vi "BuildCmdString.vi"(0 "Reply data 1":u16(ring)=1001 items=["no data"=0, "XYZ position(Command)[rad]"=1, "Joint position(Command)[rad]"=2, "Motor pulse position(Command)"=3, "XYZ position(Feedback)[rad]"=7, "Joint position(Feedback)[rad]"=8, "Motor pulse position(Feedback)"=9, "Current command[0.1%]"=10, "Current feedback[0.1%]"=11, "Robot information"=12, "Position droop"=13, "Speed(Commond)[rpm]"=14, "Speed(Feedback)[rpm]"=15, "Axis load level[%]"=16, "Encoder temperature[C]"=17, "Encoder misscount"=18, "Motor voltage[V]"=19, "Regeneration level[%]"=20, "Tolerable command+[0.1%]"=21, "Tolerable command-[0.1%]"=22, "RMS current[0.1%]"=23, "Force sensor current position"=101, "Force sensor current position(after)"=102, "Force sensor current position(before)"=103, "Position command of the force sensor correction"=104, "COL presumed torque[0.1%]"=111, "COL thershold+[0.1%]"=112, "COL thershold-[0.1%]"=113, "XYZ position(Command)[deg]"=1001, "Joint position(Command)[deg]"=1002, "XYZ position(Feedback)[deg]"=1007, "Joint position(Feedback)[deg]"=1008, "Current command[A]"=1010, "Current feedback[A]"=1011, "Tolerable command+[A]"=1012, "Tolerable command-[A]"=1013, "RMS current[A]"=1014], 1 "Input signal number":u16 max=32767, 2 "Reply data 2":u16(ring)=1002 items=["no data"=0, "XYZ position(Command)[rad]"=1, "Joint position(Command)[rad]"=2, "Motor pulse position(Command)"=3, "XYZ position(Feedback)[rad]"=7, "Joint position(Feedback)[rad]"=8, "Motor pulse position(Feedback)"=9, "Current command[0.1%]"=10, "Current feedback[0.1%]"=11, "Robot information"=12, "Position droop"=13, "Speed(Commond)[rpm]"=14, "Speed(Feedback)[rpm]"=15, "Axis load level[%]"=16, "Encoder temperature[C]"=17, "Encoder misscount"=18, "Motor voltage[V]"=19, "Regeneration level[%]"=20, "Tolerable command+[0.1%]"=21, "Tolerable command-[0.1%]"=22, "RMS current[0.1%]"=23, "Force sensor current position"=101, "Force sensor current position(after)"=102, "Force sensor current position(before)"=103, "Position command of the force sensor correction"=104, "COL presumed torque[0.1%]"=111, "COL thershold+[0.1%]"=112, "COL thershold-[0.1%]"=113, "XYZ position(Command)[deg]"=1001, "Joint position(Command)[deg]"=1002, "XYZ position(Feedback)[deg]"=1007, "Joint position(Feedback)[deg]"=1008, "Current command[A]"=1010, "Current feedback[A]"=1011, "Tolerable command+[A]"=1012, "Tolerable command-[A]"=1013, "RMS current[A]"=1014], 3 "Reply data 3":u16(ring)=102 items=["no data"=0, "XYZ position(Command)[rad]"=1, "Joint position(Command)[rad]"=2, "Motor pulse position(Command)"=3, "XYZ position(Feedback)[rad]"=7, "Joint position(Feedback)[rad]"=8, "Motor pulse position(Feedback)"=9, "Current command[0.1%]"=10, "Current feedback[0.1%]"=11, "Robot information"=12, "Position droop"=13, "Speed(Commond)[rpm]"=14, "Speed(Feedback)[rpm]"=15, "Axis load level[%]"=16, "Encoder temperature[C]"=17, "Encoder misscount"=18, "Motor voltage[V]"=19, "Regeneration level[%]"=20, "Tolerable command+[0.1%]"=21, "Tolerable command-[0.1%]"=22, "RMS current[0.1%]"=23, "Force sensor current position"=101, "Force sensor current position(after)"=102, "Force sensor current position(before)"=103, "Position command of the force sensor correction"=104, "COL presumed torque[0.1%]"=111, "COL thershold+[0.1%]"=112, "COL thershold-[0.1%]"=113, "XYZ position(Command)[deg]"=1001, "Joint position(Command)[deg]"=1002, "XYZ position(Feedback)[deg]"=1007, "Joint position(Feedback)[deg]"=1008, "Current command[A]"=1010, "Current feedback[A]"=1011, "Tolerable command+[A]"=1012, "Tolerable command-[A]"=1013, "RMS current[A]"=1014], 4 "Output signal number":u16 max=32767, 5 "Reply data 4":u16(ring)=103 items=["no data"=0, "XYZ position(Command)[rad]"=1, "Joint position(Command)[rad]"=2, "Motor pulse position(Command)"=3, "XYZ position(Feedback)[rad]"=7, "Joint position(Feedback)[rad]"=8, "Motor pulse position(Feedback)"=9, "Current command[0.1%]"=10, "Current feedback[0.1%]"=11, "Robot information"=12, "Position droop"=13, "Speed(Commond)[rpm]"=14, "Speed(Feedback)[rpm]"=15, "Axis load level[%]"=16, "Encoder temperature[C]"=17, "Encoder misscount"=18, "Motor voltage[V]"=19, "Regeneration level[%]"=20, "Tolerable command+[0.1%]"=21, "Tolerable command-[0.1%]"=22, "RMS current[0.1%]"=23, "Force sensor current position"=101, "Force sensor current position(after)"=102, "Force sensor current position(before)"=103, "Position command of the force sensor correction"=104, "COL presumed torque[0.1%]"=111, "COL thershold+[0.1%]"=112, "COL thershold-[0.1%]"=113, "XYZ position(Command)[deg]"=1001, "Joint position(Command)[deg]"=1002, "XYZ position(Feedback)[deg]"=1007, "Joint position(Feedback)[deg]"=1008, "Current command[A]"=1010, "Current feedback[A]"=1011, "Tolerable command+[A]"=1012, "Tolerable command-[A]"=1013, "RMS current[A]"=1014]) -> (7 "CMDString":string)   [LabVIEW 2018]
panel:
  in  "Command":u16(ring)=1 items=["Start"=1, "End"=255]
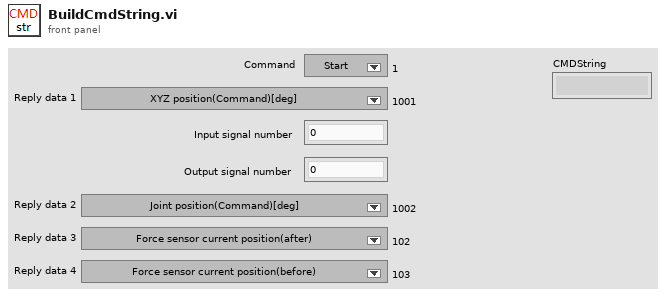
[diagram p1: front panel]
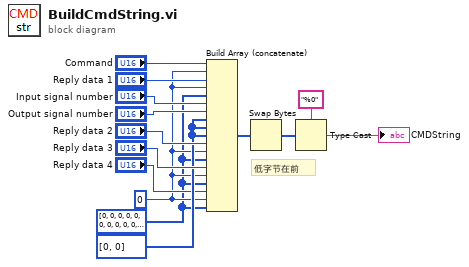
[diagram p0: block diagram]
diagram:
  w7 = u16[] [0, 0]
  w4 = u16[] [0, 0, 0, 0, 0, 0, 0, 0, 0, 0, 0, 0, 0, 0, 0, 0, 0, 0, 0, 0]
  w5 = u16 0
  # "低字节在前"
  n1 = Build Array (concatenate)("Command", w5, "Reply data 1", w5, w4, "Input signal number", "Output signal number", w7, w7, w7, "Reply data 2", w5, w4, "Reply data 3", w5, w4, "Reply data 4", w5, w4) -> (w3:u16[])
  n2 = Swap Bytes(anything=w3) -> (byte swapped=w2:u16[])
  n3 = Type Cast(type="%0" ("格式字符串"), x=w2) -> (*(type *) &x=→"CMDString":string)
